vi "Mojo.vi"(2 "Length":i16, 3 "Data In":i32[](array[numeric]), 4 "Increment":bool, 5 "Address":u32, 6 "Mode":u8(ring) items=["Open", "Close", "Read", "Write"], 7 "Port In":refnum<visa-resource-name>) -> (0 "Data Out":i32[](array[numeric]), 1 "Port Out":refnum<visa-resource-name>)   [LabVIEW 2018]
uses:
  <vilib>/Instr/_visa.llb/VISA Configure Serial Port (Instr).vi
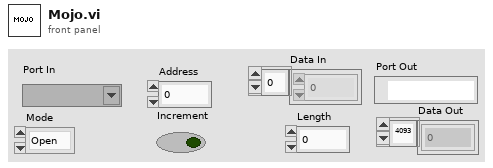
[diagram p1: front panel]
types:
  T1 = enum16{"big-endian, network order", "native, host order", "little-endian"}
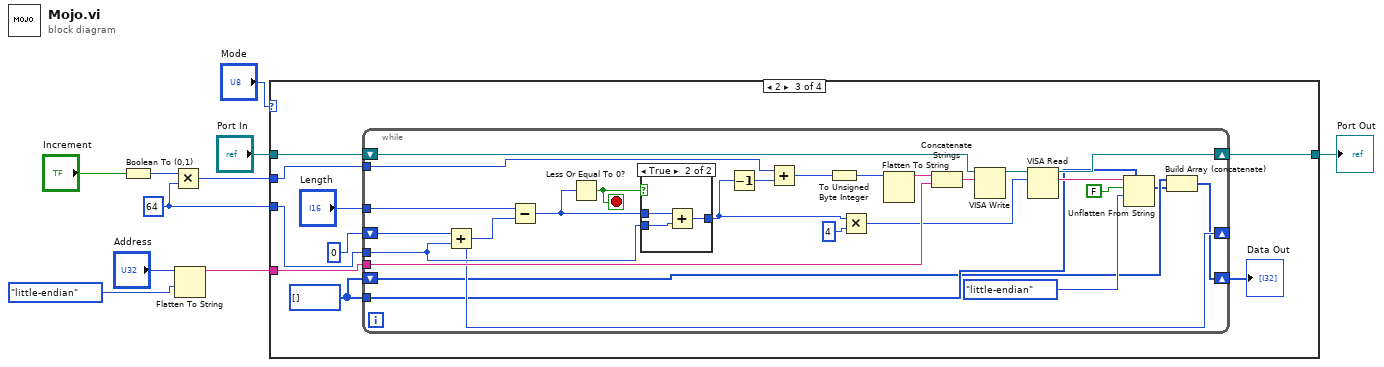
[diagram p0: block diagram]
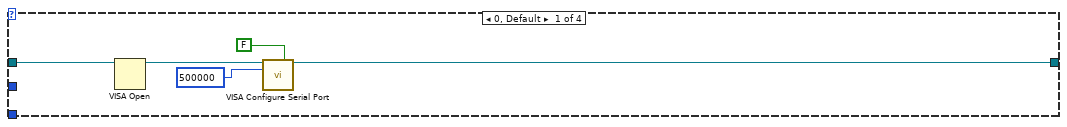
[diagram p2: hidden frame]
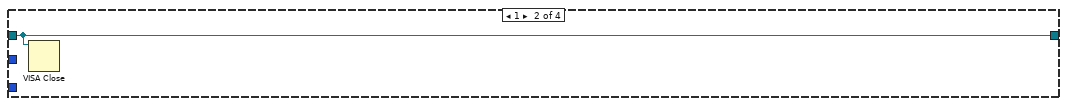
[diagram p3: hidden frame]
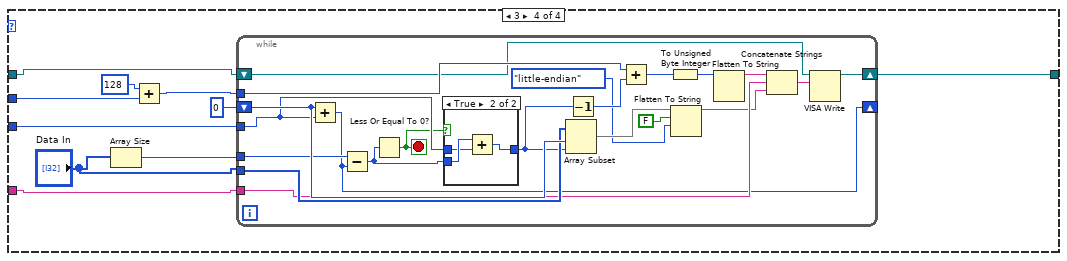
[diagram p5: hidden frame]
diagram:
  w5 = i16 64 ("y")
  n1 = Boolean To (0,1)(Boolean="Increment") -> (0, 1=w7:i16)
  n2 = Multiply(x=w7, y=w5) -> (x*y=w6:i16)
  n3 = Flatten To String(anything="Address", byte order (0:big-endian, network order)=T1."little-endian") -> (data string=w1:string)  [unwired: 2 in, 2 out]
  n4 = case shown="2" "Mode" {
    tunnel: [w11 w16 w22 w59] -> w9
    tunnel: w1 -> [_ _ w23 w60]
    tunnel: w6 -> [_ _ w19 w62]
    tunnel: w5 -> [_ _ w24 w64]
    tunnel: "Port In" -> [w13 w16 w21 w58]
    frame 0, Default {
      n5 = VISA Open(VISA resource name=w13) -> (VISA resource name=w12:refnum<visa-resource-name>)  [unwired: 4 in, 1 out]
      n6 = call-poly "VISA Configure Serial Port"("VISA resource name"=w12, "Enable Termination\nChar (T)"=FALSE ("Enable Termination\nChar (T)"), "baud rate (9600)"=u32 500000) -> ("VISA resource name out"=w11:refnum<visa-resource-name>)  [unwired: 11 in, 1 out]
    }
    frame 1 {
      n7 = VISA Close(VISA resource name=w16) -> ()  [unwired: 1 in, 1 out]
    }
    frame 2 {
      w18 = i32[] [] ("Data Out")
      n8 = while {
        shift-right: [w44] -> _
        shift-left: 0 -> [w51]
        tunnel: w24 -> [w50]
        tunnel: w19 -> [w48]
        tunnel: w23 -> [w45]
        shift-right: [w36] -> w22
        shift-left: w21 -> [w41]
        tunnel: "Length" -> [w38]
        shift-right: [w26] -> w17
        shift-left: w18 -> [w28]
        tunnel: w18 -> [w29]
        stop <- w43 stop-if-true
        n9 = Add(x=w51, y=w50) -> (x+y=w44:i32)
        n10 = Subtract(x=w38, y=w44) -> (x-y=w49:i32)
        n11 = Less Or Equal To 0?(x=w49) -> (x <= 0?=w43:bool)
        n12 = case shown="True" w43 {
          tunnel: w50 -> [w52 w53]
          tunnel: [w52 w54] -> w35
          tunnel: w49 -> [_ w55]
          frame False {
          }
          frame True {
            n13 = Add(x=w55, y=w53) -> (x+y=w54:i32)
          }
        }
        n14 = Decrement(x=w35) -> (x-1=w47:i32)
        n15 = Add(x=w48, y=w47) -> (x+y=w46:i32)
        n16 = To Unsigned Byte Integer(number=w46) -> (unsigned 8bit integer=w40:u8)
        n17 = Multiply(x=w35, y=4) -> (x*y=w33:i32)
        n18 = Flatten To String(anything=w40) -> (data string=w39:string)  [unwired: 3 in, 2 out]
        n19 = Concatenate Strings(w39, w45) -> (w42:string)
        n20 = VISA Write(VISA resource name=w41, write buffer=w42) -> (VISA resource name out=w37:refnum<visa-resource-name>)  [unwired: 1 in, 2 out]
        n21 = VISA Read(VISA resource name=w37, byte count=w33) -> (VISA resource name out=w36:refnum<visa-resource-name>, read buffer=w32:string)  [unwired: 1 in, 2 out]
        n22 = Unflatten From String(type=w29, binary string=w32, data includes array or string size? (T)=FALSE, byte order (0:big-endian, network order)=T1."little-endian") -> (value=w27:i32[])  [unwired: 1 in, 2 out]
        n23 = Build Array (concatenate)(w28, w27) -> (w26:i32[])
      }
      "Data Out" <- w17
    }
    frame 3 {
      n24 = Array Size(array="Data In") -> (size(s)=w56:i32)
      n25 = Add(x=i16 128 ("y"), y=w62) -> (x+y=w61:i16)
      n26 = while {
        shift-right: [w76] -> _
        shift-left: 0 -> [w86]
        tunnel: w64 -> [w83]
        tunnel: w56 -> [w84]
        tunnel: "Data In" -> [w85]
        tunnel: w61 -> [w81]
        tunnel: w60 -> [w77]
        shift-right: [w72] -> w59
        shift-left: w58 -> [w73]
        stop <- w75 stop-if-true
        n27 = Add(x=w86, y=w83) -> (x+y=w76:i32)
        n28 = Subtract(x=w84, y=w76) -> (x-y=w82:i32)
        n29 = Less Or Equal To 0?(x=w82) -> (x <= 0?=w75:bool)
        n30 = case shown="True" w75 {
          tunnel: w83 -> [w87 w88]
          tunnel: [w87 w89] -> w80
          tunnel: w82 -> [_ w90]
          frame False {
          }
          frame True {
            n31 = Add(x=w90, y=w88) -> (x+y=w89:i32)
          }
        }
        n32 = Array Subset(array=w85, index=w86, length=w80) -> (w71:i32[])
        n33 = Decrement(x=w80) -> (x-1=w79:i32)
        n34 = Add(x=w81, y=w79) -> (x+y=w78:i32)
        n35 = To Unsigned Byte Integer(number=w78) -> (unsigned 8bit integer=w67:u8)
        n36 = Flatten To String(anything=w71, prepend array or string size? (T)=FALSE, byte order (0:big-endian, network order)=T1."little-endian") -> (data string=w69:string)  [unwired: 1 in, 2 out]
        n37 = Flatten To String(anything=w67) -> (data string=w66:string)  [unwired: 3 in, 2 out]
        n38 = Concatenate Strings(w66, w77, w69) -> (w74:string)
        n39 = VISA Write(VISA resource name=w73, write buffer=w74) -> (VISA resource name out=w72:refnum<visa-resource-name>)  [unwired: 1 in, 2 out]
      }
    }
  }
  "Port Out" <- w9
